vi "N Field Set Text Out.vi"(1 "SetFieldCluster":T1={"rate"=0.0005, "set point"=0.0, "extra wait"=5, "wait option"=1} {"wait option" items=["Do not wait, just move on", "Wait until it reaches the set point."]; "extra wait" min=0; "set point" format="%.5f"; "rate" format="%.5f"}) -> (0 "Command text":string[][](array[string]))   [LabVIEW 2020]
uses:
  Field Set.ctl
panel:
  out "String Cluster":T2
  # "Set Field Command"
  # "T"
  # "at"
  # "T/min"
  # "1. Sweep field to"
  # "2. AND wait extra"
  # "seconds"
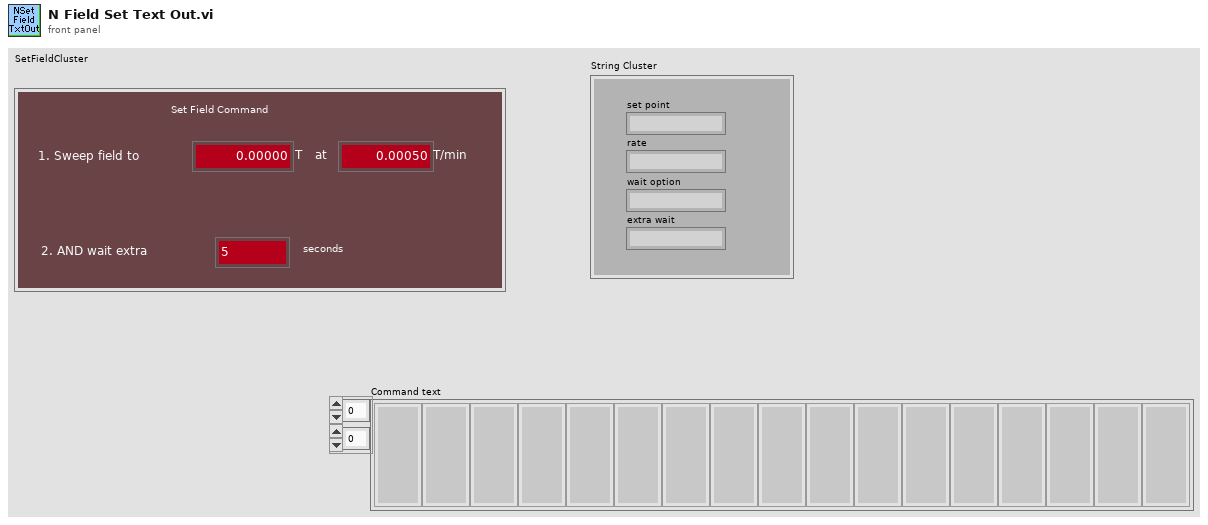
[diagram p1: front panel]
types:
  T1 = typedef "Field Set.ctl" = cluster{"rate":dbl, "set point":dbl, "extra wait":i32, "wait option":u16}
  T2 = cluster{"set point":string, "rate":string, "wait option":string, "extra wait":string}
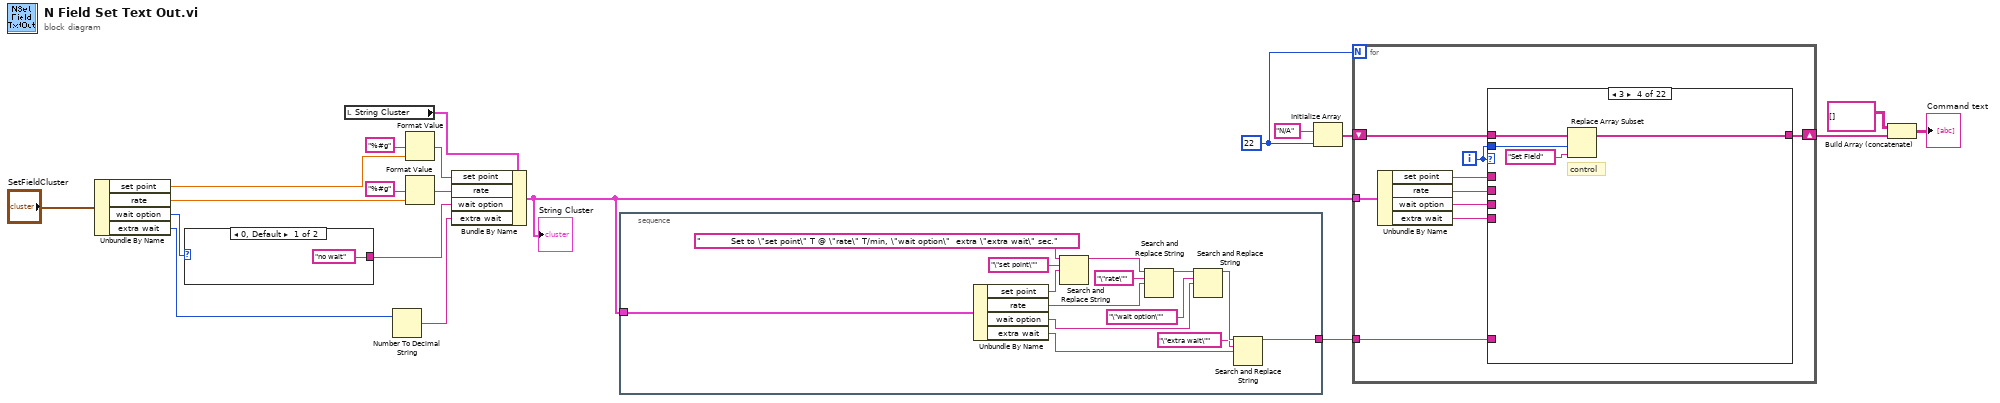
[diagram p0: block diagram]
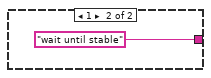
[diagram p2: hidden frame]
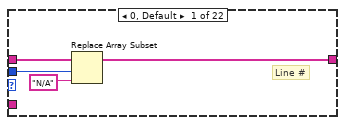
[diagram p3: hidden frame]
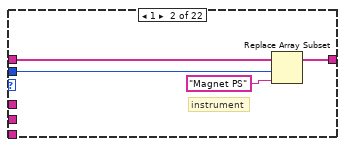
[diagram p4: hidden frame]
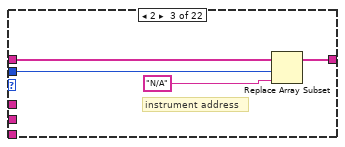
[diagram p5: hidden frame]
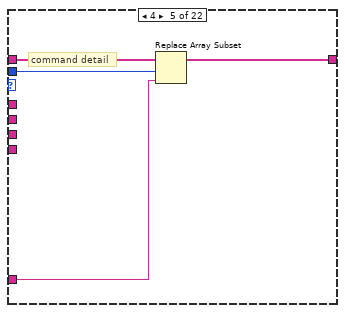
[diagram p6: hidden frame]
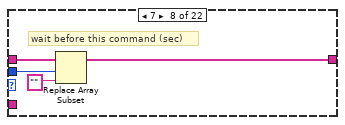
[diagram p9: hidden frame]
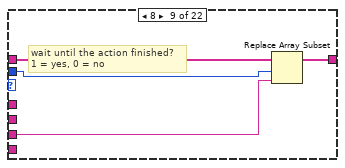
[diagram p10: hidden frame]
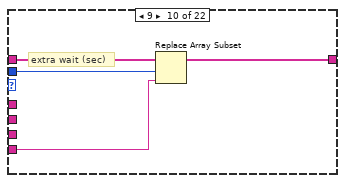
[diagram p11: hidden frame]
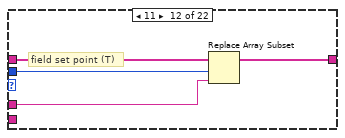
[diagram p13: hidden frame]
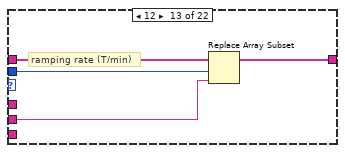
[diagram p14: hidden frame]
diagram:
  w17 = 22
  n1 = Unbundle By Name("SetFieldCluster") -> ("set point"=w14:dbl, "rate"=w13:dbl, "wait option"=w12:u16, "extra wait"=w11:i32)
  n2 = case shown="0, Default" w12 {
    tunnel: ["no wait" "wait until stable"] -> w5
    frame 0, Default {
    }
    frame 1 {
    }
  }
  n3 = local read "String Cluster"() -> (w8:T2)
  n4 = Number To Decimal String(number=w11) -> (decimal integer string=w4:string)  [unwired: 1 in]
  n5 = Format Value(format string="%#g", value (0)=w14) -> (output string=w7:string)  [unwired: 1 in]
  n6 = Format Value(format string="%#g", value (0)=w13) -> (output string=w6:string)  [unwired: 1 in]
  n7 = Bundle By Name(cluster=w8, "set point"=w7, "rate"=w6, "wait option"=w5, "extra wait"=w4) -> (w2:T2)
  "String Cluster" <- w2
  n8 = stacked-sequence {
    tunnel: [w28] -> w3
    tunnel: w2 -> [w27]
    frame #0 {
      n9 = Unbundle By Name(w27) -> ("set point"=w26:string, "rate"=w25:string, "wait option"=w24:string, "extra wait"=w23:string)
      n10 = Search and Replace String(input string="          Set to \"set point\" T @ \"rate\" T/min, \"wait option\"  extra \"extra wait\" sec.", search string="\"set point\"", replace string=w26) -> (result string=w34:string)  [unwired: 5 in, 3 out]
      n11 = Search and Replace String(input string=w34, search string="\"rate\"", replace string=w25) -> (result string=w35:string)  [unwired: 5 in, 3 out]
      n12 = Search and Replace String(input string=w35, search string="\"wait option\"", replace string=w24) -> (result string=w36:string)  [unwired: 5 in, 3 out]
      n13 = Search and Replace String(input string=w36, search string="\"extra wait\"", replace string=w23) -> (result string=w28:string)  [unwired: 5 in, 3 out]
    }
  }
  n14 = Initialize Array("N/A", w17) -> (w16:string[])
  n15 = for {
    N: w17 -> [_]
    shift-right: [w43] -> w15
    shift-left: w16 -> [w44]
    tunnel: w3 -> [w42]
    tunnel: w2 -> [w41]
    i -> [w45]
    n16 = Unbundle By Name(w41) -> ("set point"=w38:string, "rate"=w37:string, "wait option"=w40:string, "extra wait"=w39:string)
    n17 = case shown="3" w45 {
      tunnel: w45 -> [w48 w52 w56 w59 w64 _ _ w69 w73 w77 _ w82 w86 _ _ _ _ _ _ _ _ _]
      tunnel: w44 -> [w49 w51 w55 w60 w65 w66 w67 w71 w75 w79 w80 w83 w88 w89 w90 w91 w92 w93 w94 w95 w96 w97]
      tunnel: [w46 w50 w54 w58 w63 w66 w67 w70 w74 w78 w80 w84 w87 w89 w90 w91 w92 w93 w94 w95 w96 w97] -> w43
      tunnel: w42 -> [_ _ _ _ w62 _ _ _ _ _ _ _ _ _ _ _ _ _ _ _ _ _]
      tunnel: w40 -> [_ _ _ _ _ _ _ _ w72 _ _ _ _ _ _ _ _ _ _ _ _ _]
      tunnel: w39 -> [_ _ _ _ _ _ _ _ _ w76 _ _ _ _ _ _ _ _ _ _ _ _]
      tunnel: w38 -> [_ _ _ _ _ _ _ _ _ _ _ w81 _ _ _ _ _ _ _ _ _ _]
      tunnel: w37 -> [_ _ _ _ _ _ _ _ _ _ _ _ w85 _ _ _ _ _ _ _ _ _]
      frame 0, Default {
        # "Line #"
        n18 = Replace Array Subset(array=w49, new element="N/A", index=w48) -> (w46:string[])
      }
      frame 1 {
        # "instrument"
        n19 = Replace Array Subset(array=w51, new element="Magnet PS", index=w52) -> (w50:string[])
      }
      frame 2 {
        # "instrument address"
        n20 = Replace Array Subset(array=w55, new element="N/A", index=w56) -> (w54:string[])
      }
      frame 3 {
        # "control"
        n21 = Replace Array Subset(array=w60, new element="Set Field", index=w59) -> (w58:string[])
      }
      frame 4 {
        # "command detail"
        n22 = Replace Array Subset(array=w65, new element=w62, index=w64) -> (w63:string[])
      }
      frame 5 {
        # "in  case 1"
      }
      frame 6 {
        # "in case 2"
      }
      frame 7 {
        # "wait before this command (sec)"
        n23 = Replace Array Subset(array=w71, new element="" ("new element/subarray"), index=w69) -> (w70:string[])
      }
      frame 8 {
        # "wait until the action finished?\n1 = yes, 0 = no"
        n24 = Replace Array Subset(array=w75, new element=w72, index=w73) -> (w74:string[])
      }
      frame 9 {
        # "extra wait (sec)"
        n25 = Replace Array Subset(array=w79, new element=w76, index=w77) -> (w78:string[])
      }
      frame 10 {
      }
      frame 11 {
        # "field set point (T)"
        n26 = Replace Array Subset(array=w83, new element=w81, index=w82) -> (w84:string[])
      }
      frame 12 {
        # "ramping rate (T/min)"
        n27 = Replace Array Subset(array=w88, new element=w85, index=w86) -> (w87:string[])
      }
      frame 13 {
      }
      frame 14 {
      }
      frame 15 {
      }
      frame 16 {
      }
      frame 17 {
      }
      frame 18 {
      }
      frame 19 {
      }
      frame 20 {
      }
      frame 21 {
      }
    }
  }
  n28 = Build Array (concatenate)(string[][] [], w15) -> (→"Command text":string[][])
